vi "convert raw to hex.vi"(11 "String":string) -> (3 "hex integer string":string[](array[string]))   [LabVIEW 2017]
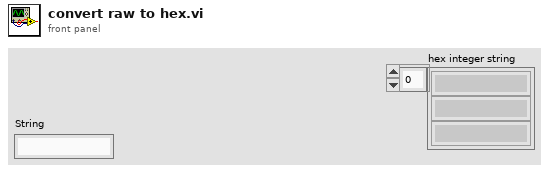
[diagram p1: front panel]
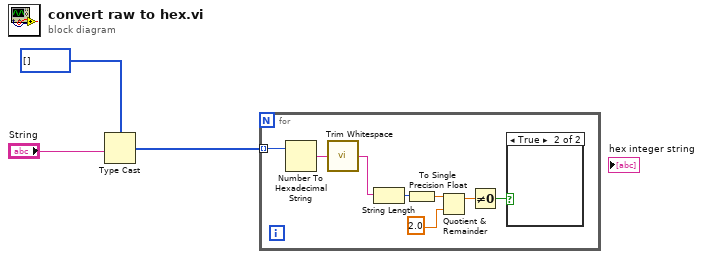
[diagram p0: block diagram]
diagram:
  n1 = Type Cast(type=u8[] [], x="String") -> (*(type *) &x=w1:u8[])
  n2 = for {
    tunnel: w1 -> [w11] mode=indexing
    n3 = Number To Hexadecimal String(2:w11) -> (0:w10:string)  [unwired: 1 in]
    n4 = call <vilib>:"Trim Whitespace.vi"("string"=w10) -> ("trimmed string"=w9:string)  [unwired: 1 in]
    n5 = String Length(string=w9) -> (length=w8:i32)
    n6 = To Single Precision Float(number=w8) -> (single precision float=w7:sgl)
    n7 = Quotient & Remainder(x=w7, y=sgl 2.0) -> (x-y*floor(x/y)=w5:sgl)  [unwired: 1 out]
    n8 = Not Equal To 0?(x=w5) -> (x != 0?=w4:bool)
    n9 = case shown="True" w4 {
      frame False {
      }
      frame True {
      }
    }
  }
